vi "wait.vi"(0 "Wait (s)":dbl) -> (1 "Done":bool, 2 "Wait Time\nRemaining":string)   [LabVIEW 2011]
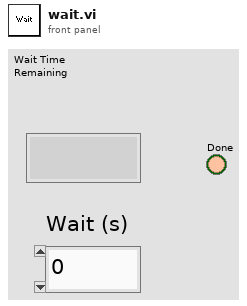
[diagram p1: front panel]
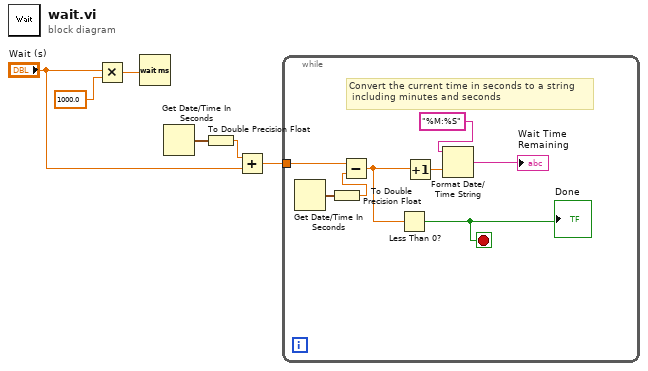
[diagram p0: block diagram]
diagram:
  n1 = Multiply(x="Wait (s)", y=1000.0) -> (x*y=w3:dbl)
  n2 = Wait (ms)(milliseconds to wait=w3) -> ()  [unwired: 1 out]
  n3 = Get Date/Time In Seconds() -> (seconds since 1Jan1904=w4:timestamp)
  n4 = To Double Precision Float(number=w4) -> (double precision float=w5:dbl)
  n5 = Add(x=w5, y="Wait (s)") -> (x+y=w2:dbl)
  n6 = while {
    tunnel: w2 -> [w11]
    stop <- w8 stop-if-true
    # "Convert the current time in seconds to a string\n including minutes and seconds"
    n7 = Get Date/Time In Seconds() -> (seconds since 1Jan1904=w12:timestamp)
    n8 = To Double Precision Float(number=w12) -> (double precision float=w13:dbl)
    n9 = Subtract(x=w11, y=w13) -> (x-y=w10:dbl)
    n10 = Less Than 0?(x=w10) -> (x < 0?=w8:bool)
    "Done" <- w8
    n11 = Increment(x=w10) -> (x+1=w9:dbl)
    n12 = Format Date/Time String(time format string (%c)="%M:%S", seconds (now)=w9) -> (date/time string=→"Wait Time\nRemaining":string)  [unwired: 1 out]
  }
